vi "Init Info Services.vi"(8 "error in (no error)":errorcluster, 11 "Vecto in":refnum<class "Vecto.lvclass">) -> (0 "error out":errorcluster, 3 "Vecto out":refnum<class "Vecto.lvclass">)   [LabVIEW 2020, in "Vecto.lvlib" / "Vecto.lvclass"]
uses:
  Vecto.lvclass
  Vecto.lvclass/Vecto.ctl
  InfoService/NodeStatus.lvclass
  VectoService/VectoInfo.lvclass
  Event Level.ctl
  Vecto.lvlib
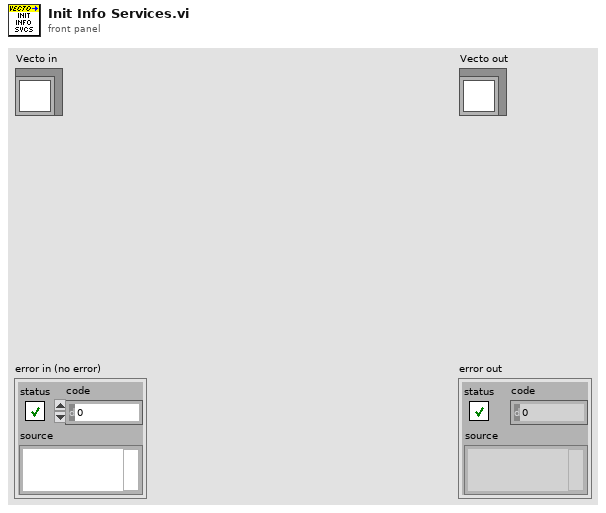
[diagram p1: front panel]
types:
  T1 = typedef "Vecto.lvlib/Event Level.ctl" = enum16{"Debug", "Info", "Warning", "Error"}
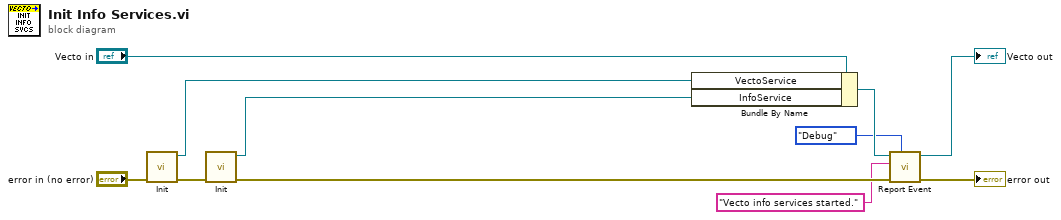
[diagram p0: block diagram]
diagram:
  n1 = call "Init.vi"("error in (no error)"="error in (no error)") -> ("error out"=w11:errorcluster, "VectoService out"=w7:refnum<class "VectoInfo.lvclass">)  [unwired: 9 in]
  n2 = call "Init.vi"("error in (no error)"=w11) -> ("error out"=w9:errorcluster, "InfoService out"=w6:refnum<class "NodeStatus.lvclass">)  [unwired: 9 in]
  n3 = Bundle By Name(cluster="Vecto in", "VectoService"=w7, "InfoService"=w6) -> (w4:refnum<class "Vecto.lvclass">)
  n4 = call "Report Event.vi"("Event Level (Info)"=Event_Level."Debug", "error in (no error)"=w9, "Message"="Vecto info services started.", "Vecto in"=w4) -> ("error out"=→"error out":errorcluster, "Vecto out"=→"Vecto out":refnum<class "Vecto.lvclass">)  [unwired: 6 in]
